vi "MeasurementInitializeVer8.0.vi"(5 "Instruments Configs In 2D array":string[][](table) caption="Instruments Configs", 7 "error in":errorcluster) -> (3 "error out":errorcluster, 4 "InstTitleNameArray":string[](array[string]))   [LabVIEW 2012]
doc: "Clear selected GPIB device and initialized selected device\nInstruments Configs In 2D array:\n0: Instrument name\n1: GPIB Address\n2: Initialized CMD\n3: Unit factor\n4: Title name\n5: Read Data CMD\n6: Info"
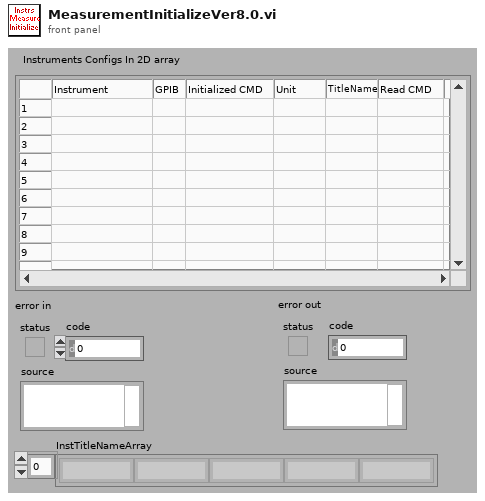
[diagram p1: front panel]
types:
  T1 = enum16{"Instrument", "Function", "GPIB", "Initiralized CMD", "Title Name", "Unit", "Read CMD", "Post CMD", "Info", "Terminator Mode"}
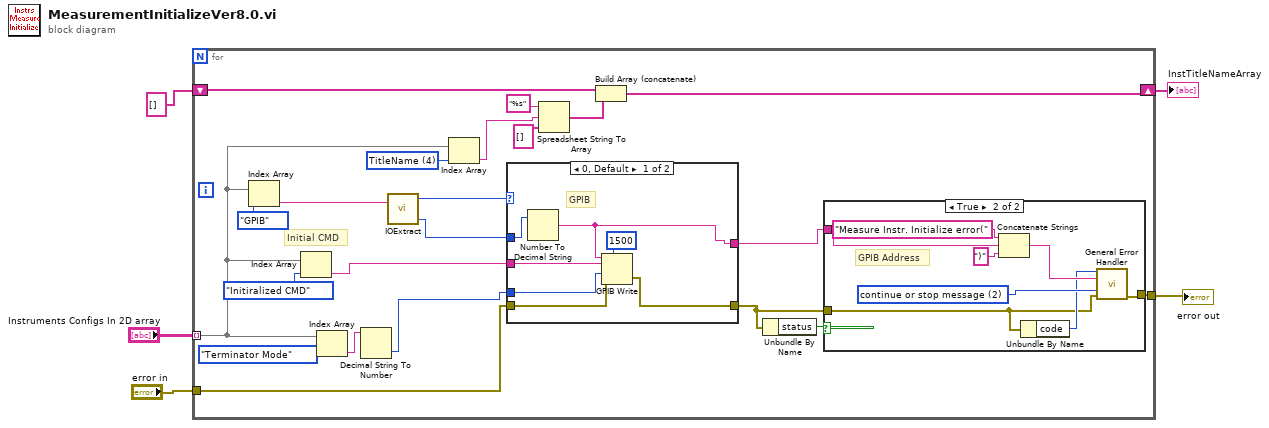
[diagram p0: block diagram]
diagram:
  n1 = for {
    tunnel: "Instruments Configs In 2D array" -> [w8] mode=indexing
    tunnel: "error in" -> [w19]
    tunnel: [w26] -> w3
    shift-right: [w6] -> w1
    shift-left: string[] [] ("Array 2") -> [w7]
    w10 = u16 4 items=["Instrument", "Function", "GPIB", "InitializedCMD", "TitleName", "Unit", "ReadCMD", "PostCMD", "Info", "Mode"] ("Ring")
    # "Initial CMD"
    n2 = Index Array(array=w8, index=T1."GPIB") -> (element=w16:string)
    n3 = Index Array(array=w8, index=T1."Initiralized CMD") -> (element=w21:string)
    n4 = Index Array(array=w8, index=T1."Terminator Mode") -> (element=w22:string)
    n5 = Decimal String To Number(string=w22) -> (number=w20:i32)  [unwired: 2 in, 1 out]
    n6 = call "IOExtract.vi"("Instrument(String)"=w16) -> ("InterfaceCode:\n0: GPIB\n1: ISOBUS"=w15:i32, "Address"=w14:i32)  [unwired: 1 in, 1 out]
    n7 = Index Array(array=w8, index=w10) -> (element=w9:string)
    n8 = case shown="0, Default" w15 {
      tunnel: w14 -> [w30 _]
      tunnel: w21 -> [w31 w35]
      tunnel: w20 -> [w32 _]
      tunnel: w19 -> [w34 w36]
      tunnel: [w33 w36] -> w18
      tunnel: [w29 w35] -> w17
      frame 0, Default {
        # "GPIB"
        n9 = Number To Decimal String(number=w30) -> (decimal integer string=w29:string)  [unwired: 1 in]
        n10 = GPIB Write(0:w29, 1:w31, 2:w32, 3:w34, 4:1500 ("timeout ms (488.2 global)")) -> (6:w33:errorcluster)  [unwired: 1 out]
      }
      frame 1 {
        # "ISOBUS"
      }
    }
    n11 = Spreadsheet String To Array(format string="%s", spreadsheet string=w9, array type (2D Dbl)=string[] [] ("Array 2")) -> (array=w11:string[])  [unwired: 1 in]
    n12 = Build Array (concatenate)(w7, w11) -> (w6:string[])
    n13 = Unbundle By Name(w18) -> ("status"=w27:bool)
    n14 = case shown="True" w27 {
      tunnel: w18 -> [w37 w38]
      tunnel: [w37 w44] -> w26
      tunnel: w17 -> [_ w43]
      frame False {
      }
      frame True {
        w45 = 2 items=["no dialog", "OK message", "continue or stop message"] ("type of dialog (OK msg:1)")
        # "GPIB Address"
        n15 = Concatenate Strings("Measure Instr. Initialize error(" ("Function"), w43, ")" ("string")) -> (w41:string)
        n16 = Unbundle By Name(w38) -> ("code"=w39:i32)
        n17 = call <vilib>:"General Error Handler.vi"("[error code] (0)"=w39, "[error source] (\" \")"=w41, "type of dialog (OK msg:1)"=w45, "error in (no error)"=w38) -> ("error out"=w44:errorcluster)  [unwired: 7 in, 4 out]
      }
    }
  }
  "error out" <- w3
  "InstTitleNameArray" <- w1
